vi "(SubVI) Theme color.vi"(1 "Classify text":string) -> (0 "Classify color":u32)   [LabVIEW 2022 SP3]
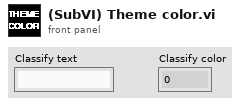
[diagram p1: front panel]
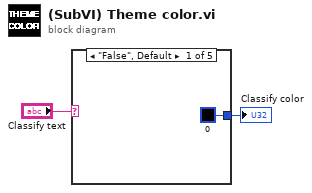
[diagram p0: block diagram]
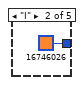
[diagram p2: hidden frame]
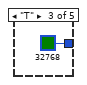
[diagram p3: hidden frame]
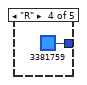
[diagram p4: hidden frame]
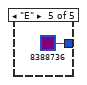
[diagram p5: hidden frame]
diagram:
  n1 = case shown="\"False\", Default" "Classify text" {
    tunnel: [u32 0 ("Classify color") u32 16746026 ("Classify color") u32 32768 ("Classify color") u32 3381759 ("Classify color") u32 8388736 ("Classify color")] -> w2
    frame "False", Default {
    }
    frame "I" {
    }
    frame "T" {
    }
    frame "R" {
    }
    frame "E" {
    }
  }
  "Classify color" <- w2
